vi "Frameremap_raw.vi"(10 "Frame Origin (m)":cluster{"Xc":sgl, "Yc":sgl} {"Yc" format="%.2p"; "Xc" format="%.2p"}, 11 "Frame Size (m)":cluster{"Width":sgl, "Height":sgl} {"Height" format="%.2p"; "Width" format="%.2p"}) -> (0 "FH (nm)":dbl, 1 "FW (nm)":dbl, 2 "Z Origin (nm)":dbl, 3 "X Origin (nm)":dbl)   [LabVIEW 2019]
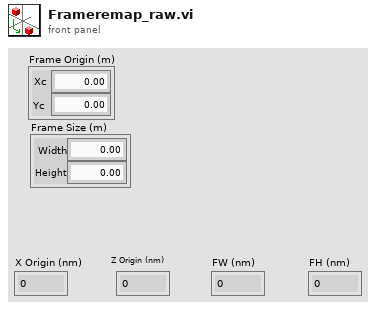
[diagram p1: front panel]
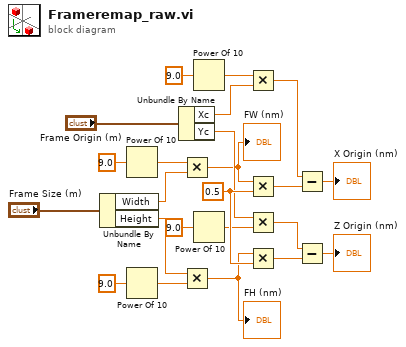
[diagram p0: block diagram]
diagram:
  w23 = 0.5 ("y")
  n1 = Unbundle By Name("Frame Size (m)") -> ("Width"=w15:sgl, "Height"=w12:sgl)
  n2 = Power Of 10(x=9.0) -> (10^x=w16:dbl)
  n3 = Power Of 10(x=9.0) -> (10^x=w14:dbl)
  n4 = Unbundle By Name("Frame Origin (m)") -> ("Xc"=w6:sgl, "Yc"=w5:sgl)
  n5 = Multiply(x=w16, y=w15) -> (x*y=w2:dbl)
  "FW (nm)" <- w2
  n6 = Multiply(x=w12, y=w14) -> (x*y=w1:dbl)
  "FH (nm)" <- w1
  n7 = Power Of 10(x=9.0) -> (10^x=w9:dbl)
  n8 = Power Of 10(x=9.0) -> (10^x=w8:dbl)
  n9 = Multiply(x=w9, y=w6) -> (x*y=w4:dbl)
  n10 = Multiply(x=w2, y=w23) -> (x*y=w22:dbl)
  n11 = Multiply(x=w5, y=w8) -> (x*y=w3:dbl)
  n12 = Multiply(x=w1, y=w23) -> (x*y=w21:dbl)
  n13 = Subtract(x=w4, y=w22) -> (x-y=→"X Origin (nm)":dbl)
  n14 = Subtract(x=w3, y=w21) -> (x-y=→"Z Origin (nm)":dbl)
